vi "LVMark_Apply_Properties.vi"(8 "error in":errorcluster, 9 "Operations":T1[](array[typedef]), 10 "ML string":string, 11 "Text ref in":refnum<vi>) -> (0 "error out":errorcluster, 3 "Text ref out":refnum<vi>)   [LabVIEW 2009]
doc: "Applies text properties in the operations list to the referenced text control."
uses:
  LVMark_opcluster.ctl
  LVMark_optype.ctl
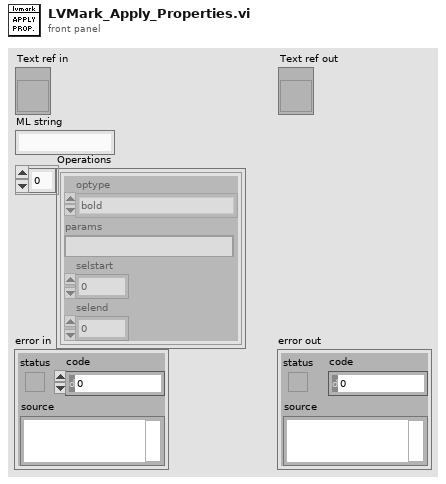
[diagram p1: front panel]
types:
  T1 = typedef "LVMark_opcluster.ctl" = cluster{"optype":T2, "params":string, "selstart":i32, "selend":i32}
  T2 = typedef "LVMark_optype.ctl" = enum16{"bold", "italic", "underline", "color", "font", "fontsize", "strikethrough"}
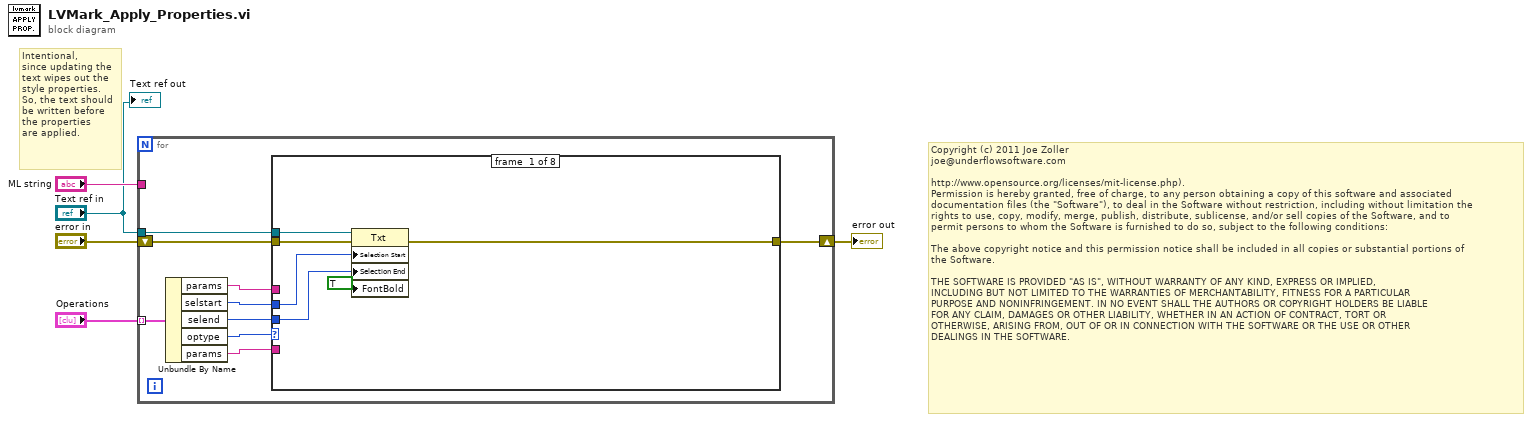
[diagram p0: block diagram]
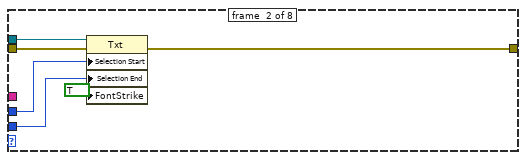
[diagram p2: hidden frame]
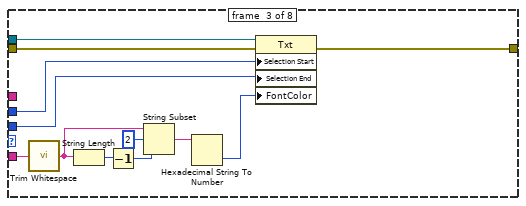
[diagram p3: hidden frame]
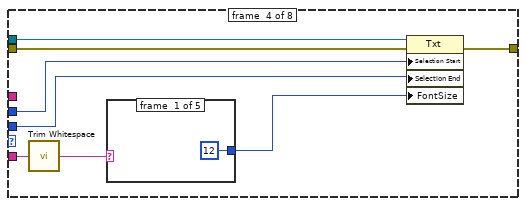
[diagram p4: hidden frame]
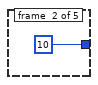
[diagram p5: hidden frame]
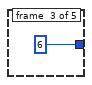
[diagram p6: hidden frame]
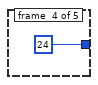
[diagram p7: hidden frame]
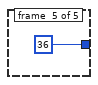
[diagram p8: hidden frame]
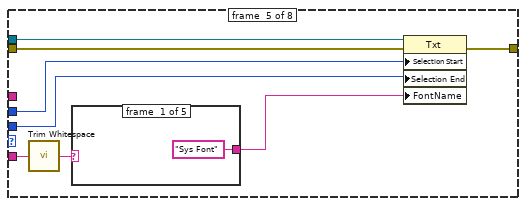
[diagram p9: hidden frame]
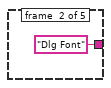
[diagram p10: hidden frame]
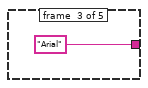
[diagram p11: hidden frame]
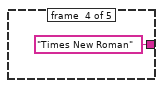
[diagram p12: hidden frame]
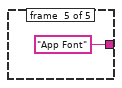
[diagram p13: hidden frame]
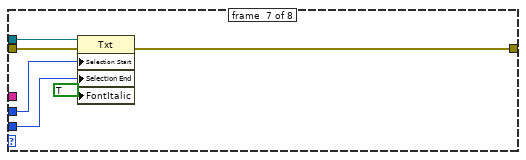
[diagram p15: hidden frame]
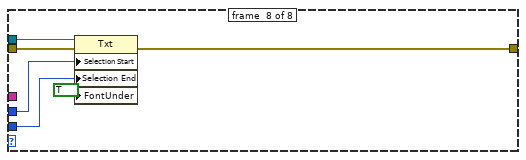
[diagram p16: hidden frame]
diagram:
  # "Copyright (c) 2011 Joe Zoller\njoe@underflowsoftware.com\n\nhttp://www.opensource.org/licenses/mit-license.php).\nPermission is hereby granted, free of charge, to any person obtaining a copy of this software and associated\ndocumentation files (the \"Software\"), to deal in the Software without restriction, including without limitation the\nrights to use, copy, modify, merge, publish, distribute, sublicense, and/or sell copies of the Software, and to\npermit persons to whom the Software is furnished to do so, subject to the following conditions:\n\nThe above copyright notice and this permission notice shall be included in all copies or substantial portions of\nthe Software.\n\nTHE SOFTWARE IS PROVIDED \"AS IS\", WITHOUT WARRANTY OF ANY KIND, EXPRESS OR IMPLIED,\nINCLUDING BUT NOT LIMITED TO THE WARRANTIES OF MERCHANTABILITY, FITNESS FOR A PARTICULAR\nPURPOSE AND NONINFRINGEMENT. IN NO EVENT SHALL THE AUTHORS OR COPYRIGHT HOLDERS BE LIABLE\nFOR ANY CLAIM, DAMAGES OR OTHER LIABILITY, WHETHER IN AN ACTION OF CONTRACT, TORT OR\nOTHERWISE, ARISING FROM, OUT OF OR IN CONNECTION WITH THE SOFTWARE OR THE USE OR OTHER\nDEALINGS IN THE SOFTWARE."
  # "Intentional,\nsince updating the\ntext wipes out the\nstyle properties.\nSo, the text should\nbe written before\nthe properties\nare applied."
  n1 = for {
    tunnel: "Text ref in" -> [w14]
    shift-right: [w12] -> w2
    shift-left: "error in" -> [w13]
    tunnel: "Operations" -> [w11] mode=indexing
    tunnel: "ML string" -> [_]
    n2 = Unbundle By Name(w11) -> ("params"=w7:string, "selstart"=w9:i32, "selend"=w8:i32, "optype"=w10:T2, "params"=w6:string)
    n3 = case shown="\"fontsize\"" w10 {
      tunnel: w14 -> [w20 w26 w36 w44 w57 _ w71 w77]
      tunnel: w9 -> [w19 w25 w32 w42 w55 _ w70 w76]
      tunnel: w8 -> [w18 w24 w31 w41 w54 _ w69 w75]
      tunnel: w13 -> [w16 w22 w38 w46 w59 w65 w67 w73]
      tunnel: [w15 w21 w37 w45 w58 w65 w66 w72] -> w12
      tunnel: w7 -> [_ _ _ _ _ _ _ _]
      tunnel: w6 -> [_ _ w34 w43 w56 _ _ _]
      frame #0 {
        n4 = property class="Txt"(reference=w20, error in=w16, "Selection Start"=w19, "Selection End"=w18, "FontBold"=TRUE ("Font:Bold")) -> (error out=w15:errorcluster)  [unwired: 1 out]
      }
      frame #1 {
        n5 = property class="Txt"(reference=w26, error in=w22, "Selection Start"=w25, "Selection End"=w24, "FontStrike"=TRUE ("Font:Bold")) -> (error out=w21:errorcluster)  [unwired: 1 out]
      }
      frame #2 {
        n6 = call <vilib>:"Trim Whitespace.vi"("string"=w34) -> ("trimmed string"=w33:string)  [unwired: 1 in]
        n7 = String Length(string=w33) -> (length=w29:i32)
        n8 = Decrement(x=w29) -> (x-1=w28:i32)
        n9 = String Subset(string=w33, offset (0)=2, length (rest)=w28) -> (substring=w27:string)
        n10 = Hexadecimal String To Number(string=w27) -> (number=w35:u32)  [unwired: 2 in, 1 out]
        n11 = property class="Txt"(reference=w36, error in=w38, "Selection Start"=w32, "Selection End"=w31, "FontColor"=w35) -> (error out=w37:errorcluster)  [unwired: 1 out]
      }
      frame #3 {
        n12 = call <vilib>:"Trim Whitespace.vi"("string"=w43) -> ("trimmed string"=w40:string)  [unwired: 1 in]
        n13 = case shown="\"[small]\"" w40 {
          tunnel: [u32 12 ("Font:Size") u32 10 ("Font:Size") u32 6 ("Font:Size") u32 24 ("Font:Size") u32 36 ("Font:Size")] -> w39
          frame #0 {
          }
          frame #1 {
          }
          frame #2 {
          }
          frame #3 {
          }
          frame #4 {
          }
        }
        n14 = property class="Txt"(reference=w44, error in=w46, "Selection Start"=w42, "Selection End"=w41, "FontSize"=w39) -> (error out=w45:errorcluster)  [unwired: 1 out]
      }
      frame #4 {
        n15 = call <vilib>:"Trim Whitespace.vi"("string"=w56) -> ("trimmed string"=w53:string)  [unwired: 1 in]
        n16 = case shown="\"[App]\", Default" w53 {
          tunnel: ["Sys Font" "Dlg Font" "Arial" "Times New Roman" "App Font"] -> w52
          frame #0 {
          }
          frame #1 {
          }
          frame #2 {
          }
          frame #3 {
          }
          frame #4 {
          }
        }
        n17 = property class="Txt"(reference=w57, error in=w59, "Selection Start"=w55, "Selection End"=w54, "FontName"=w52) -> (error out=w58:errorcluster)  [unwired: 1 out]
      }
      frame #5 {
      }
      frame #6 {
        n18 = property class="Txt"(reference=w71, error in=w67, "Selection Start"=w70, "Selection End"=w69, "FontItalic"=TRUE ("Font:Italic")) -> (error out=w66:errorcluster)  [unwired: 1 out]
      }
      frame #7 {
        n19 = property class="Txt"(reference=w77, error in=w73, "Selection Start"=w76, "Selection End"=w75, "FontUnder"=TRUE ("Font:Italic")) -> (error out=w72:errorcluster)  [unwired: 1 out]
      }
    }
  }
  "error out" <- w2
  "Text ref out" <- "Text ref in"
